vi "Check if Connection Allowed.vi"(8 "error in (no error)":errorcluster, 11 "TCP slave in":refnum<class "TCP Slave.lvclass">) -> (0 "error out":errorcluster, 2 "connection allowed":bool, 3 "TCP slave out":refnum<class "TCP Slave.lvclass">)   [LabVIEW 2018, in "SubVIs.lvlib" / "TCP Slave.lvclass"]
doc: "Checks to see if a new connection is allowed."
uses:
  TCP Slave.lvclass
  TCP Slave.lvclass/TCP Slave.ctl
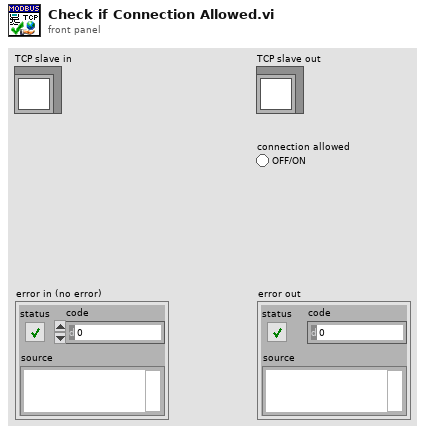
[diagram p1: front panel]
types:
  T1 = typedef "SubVIs.lvlib/TCP Slave.lvclass/Connection Counter.ctl" = cluster{"Currently Connected":u32, "Connection Records":refnum<data-value>[]}
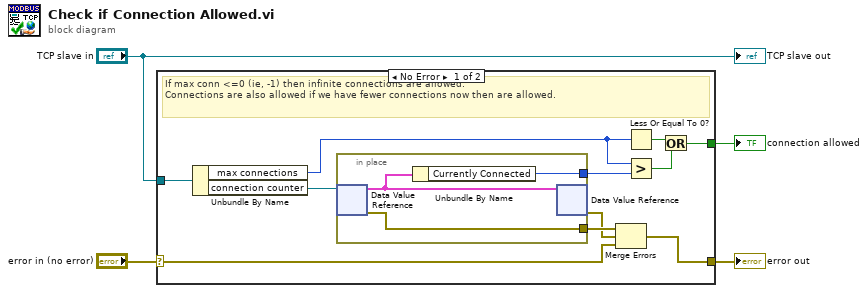
[diagram p0: block diagram]
diagram:
  n1 = case shown="No Error" "error in (no error)" {
    selector: "error in (no error)" -> [w6 w19]
    tunnel: "TCP slave in" -> [w15 _]
    tunnel: [w14 w19] -> w3
    tunnel: [w13 _] -> w2
    frame No Error {
      # "If max conn <=0 (ie, -1) then infinite connections are allowed.\nConnections are also allowed if we have fewer connections now then are allowed."
      n2 = Unbundle By Name(w15) -> ("max connections"=w7:i32, "connection counter"=w12:refnum<data-value>)
      n3 = in-place {
        in-place-border: [w17] -> w9
        in-place-border: [w16] -> w11
        n4 = in-place-dvr #1(w12) -> (w18:T1, w16:errorcluster)
        n5 = Unbundle By Name(w18) -> ("Currently Connected"=w17:u32)
        n6 = in-place-dvr #1(w18) -> (w5:errorcluster)  [unwired: 1 out]
      }
      n7 = Merge Errors(w11, w5, w6) -> (w14:errorcluster)
      n8 = Less Or Equal To 0?(x=w7) -> (x <= 0?=w10:bool)
      n9 = Greater?(x=w7, y=w9) -> (0:w8:bool)
      n10 = Or(x=w10, y=w8) -> (x .or. y?=w13:bool)
    }
    frame Error {
    }
  }
  "error out" <- w3
  "connection allowed" <- w2
  "TCP slave out" <- "TCP slave in"
